vi "Main.vi"   [LabVIEW 2021]
uses:
  <vilib>/AppBuilder/AB_API_Simple/NI_App_Builder_API.lvlib
  Builder/Builder.lvclass
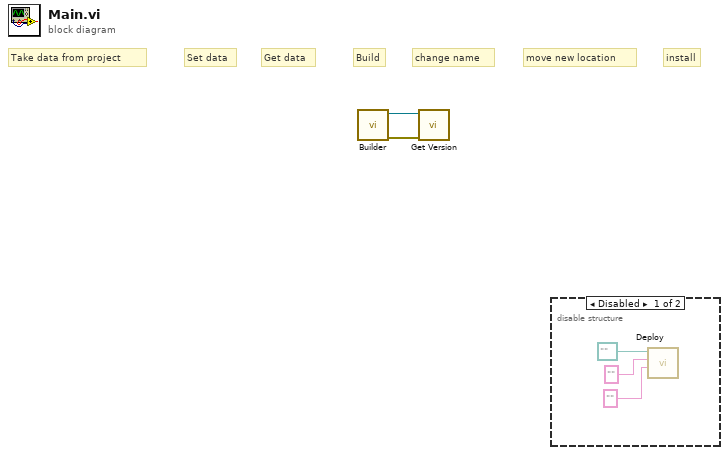
[diagram p0: block diagram]
diagram:
  # "install"
  # "move new location"
  # "change name"
  # "Build"
  # "Get data"
  # "Set data"
  # "Take data from project"
  n1 = call "Builder.vi"() -> ("error out"=w1:errorcluster, "Builder out"=w2:refnum<class "Builder.lvclass">)  [unwired: 9 in, 1 out]
  n2 = call-dynamic "Get Version.vi"("error in (no error)"=w1, "Builder in"=w2) -> ()  [unwired: 7 in, 3 out]
  n3 = disable-structure shown="Disabled" {
    frame Disabled {
      n4 = call <vilib>:"Deploy.vi"("Name of target"="", "Name of build specification (if empty: deploy all)"="", "Path to project"=path "") -> ()  [unwired: 8 in, 1 out]
    }
    frame Enabled {
    }
  }
